vi "Tosca-Execute Schedule Order Script.vi"(0 "Path":path, 11 "error in (no error)":errorcluster) -> (8 "order":i32[](array[numeric]), 15 "error out":errorcluster)   [LabVIEW 2020]
panel:
  out "Message":string
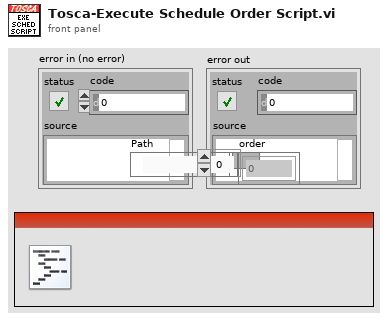
[diagram p1: front panel]
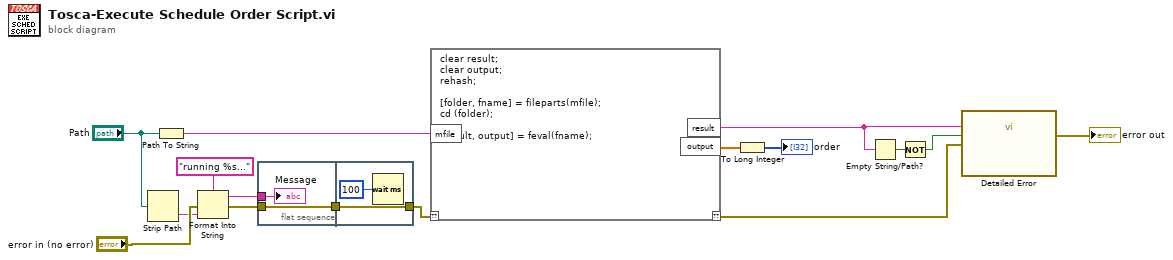
[diagram p0: block diagram]
diagram:
  n1 = Strip Path(path="Path") -> (name=w14:string)  [unwired: 1 out]
  n2 = Path To String(path="Path") -> (string=w9:string)
  n3 = Format Into String(format string="running %s...", error in="error in (no error)", w14) -> (resulting string=w13:string, error out=w12:errorcluster)  [unwired: 1 in]
  n4 = flat-sequence {
    tunnel: w13 -> [w18]
    tunnel: w12 -> [w17]
    tunnel: [w17] -> w11
    tunnel: w11 -> [w20]
    tunnel: [w20] -> w8
    frame #0 {
      "Message" <- w18
    }
    frame #1 {
      n5 = Wait (ms)(milliseconds to wait=u32 100) -> ()  [unwired: 1 out]
    }
  }
  n6 = script code="clear result;\nclear output;\nrehash;\n\n[folder, fname] = fileparts(mfile);\ncd (folder);\n\n[result, output] = feval(fname);"("??"=w8, "mfile"=w9) -> ("??"=w5:errorcluster, "result"=w3:string, "output"=w7:dbl[])
  n7 = To Long Integer(number=w7) -> (32bit integer=→"order":i32[])
  n8 = Empty String/Path?(string/path=w3) -> (empty?=w2:bool)
  n9 = Not(x=w2) -> (.not. x?=w1:bool)
  n10 = call "Detailed Error"("Details"=w3, "Error?"=w1, "Primary"=w5) -> ("detailed error"=→"error out":errorcluster)  [unwired: 12 in]
